vi "Configure All.vi"(8 "error in":errorcluster, 11 "ActorMeter in":refnum<class "ActorMeter.lvclass">) -> (0 "error out":errorcluster, 3 "ActorMeter out":refnum<class "ActorMeter.lvclass">)   [LabVIEW 2014]
uses:
  Implementations/Collector/AverageCollector1D/AverageCollector1D.lvclass
  Implementations/Extractor/MassSpectrumExtractor/MassSpectrumExtractor.lvclass
  <vilib>/ActorFramework/Actor/Actor.lvclass
  StorageService/StorageService.lvclass
  <vilib>/ActorFramework/Message/Message.lvclass
  <vilib>/ActorFramework/Message Enqueuer/Message Enqueuer.lvclass
  Model/Data/MessageToSend.ctl
  ExperimentService/ExperimentService Messages/Set Next Parameter Msg/Set Next Parameter Msg.lvclass
  ExperimentService/ExperimentService.lvclass
  StorageService/StorageService Messages/Register Msg/Register Msg.lvclass
  Model/ReplayData Msg/ReplayData Msg.lvclass
  Hardware/ParameterDevice/ParameterDevice Messages/Get Parameter Msg/Get Parameter Msg.lvclass
  StorageService/StorageService Messages/Notify All Objects Msg/Notify All Objects Msg.lvclass
  ExperimentService/ExperimentService Messages/Write StorageService Msg/Write StorageService Msg.lvclass
  Interfaces/Observable Actor/Observable Actor.lvclass
  Interfaces/Observable Actor/Observable Actor Messages/Add On Event Message Msg/Add On Event Message Msg.lvclass
  Interfaces/Observable Actor/Read Data Msg/Read Data Msg.lvclass
  <vilib>/ActorFramework/Message Enqueuer/Message Priority.ctl
  Implementations/Hardware/Simulated Hardware/ReadoutDevice/Simulated Oscilloscope/Simulated Oscilloscope.lvclass
  Implementations/Hardware/Real Hardware/ReadoutDevice/Agilent DSO-X 3032A/Agilent DSO-X 3032A.lvclass
  <vilib>/Utility/sysdir.llb/System Directory Type.ctl
  Processor/AbstractProcessor1D/AbstractProcessor1D.lvclass
  Implementations/Hardware/Simulated Hardware/ReadoutDevice/Simulated Videocamera/Simulated Videocamera.lvclass
  Implementations/Hardware/Simulated Hardware/ParameterDevice/Simulated ParameterDevice/Simulated ParameterDevice.lvclass
  Processor/AbstractProcessor2D/AbstractProcessor2D.lvclass
  Implementations/Collector/AverageCollector2D/AverageCollector2D.lvclass
  Implementations/Extractor/ImagingExtractor/ImagingExtractor.lvclass
  Extractor/AbstractExtractor/AbstractExtractor.lvclass
  Implementations/Hardware/Real Hardware/ReadoutDevice/Videoscan/Videoscan.lvclass
  SimpleExperimentService/SimpleExperimentService.lvclass
  Implementations/Hardware/Real Hardware/ParameterDevice/SolarSystems M266/SolarSystems M266.lvclass
  Implementations/Hardware/Real Hardware/ParameterDevice/Stepper3D/Stepper3D.lvclass
  ActorMeter.lvclass
  Implementations/Hardware/Real Hardware/ParameterDevice/SolarSystems M266 Old/SolarSystems M266 Old.lvclass
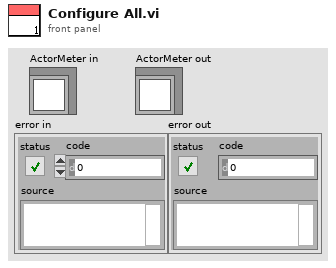
[diagram p1: front panel]
types:
  T1 = typedef "MessageToSend.ctl" = cluster{"Enqueuer":refnum<class "Message Enqueuer.lvclass">, "Message":refnum<class "Message.lvclass">}
  T2 = cluster{"Enqueuer":refnum<class "Message Enqueuer.lvclass">, "Message":refnum<class "ReplayData Msg.lvclass">}
  T3 = typedef "Actor Framework.lvlib/Message Enqueuer.lvclass/Message Priority.ctl" = enum16{"Low", "Normal", "High"}
  T4 = typedef "System Directory Type.ctl" = i32
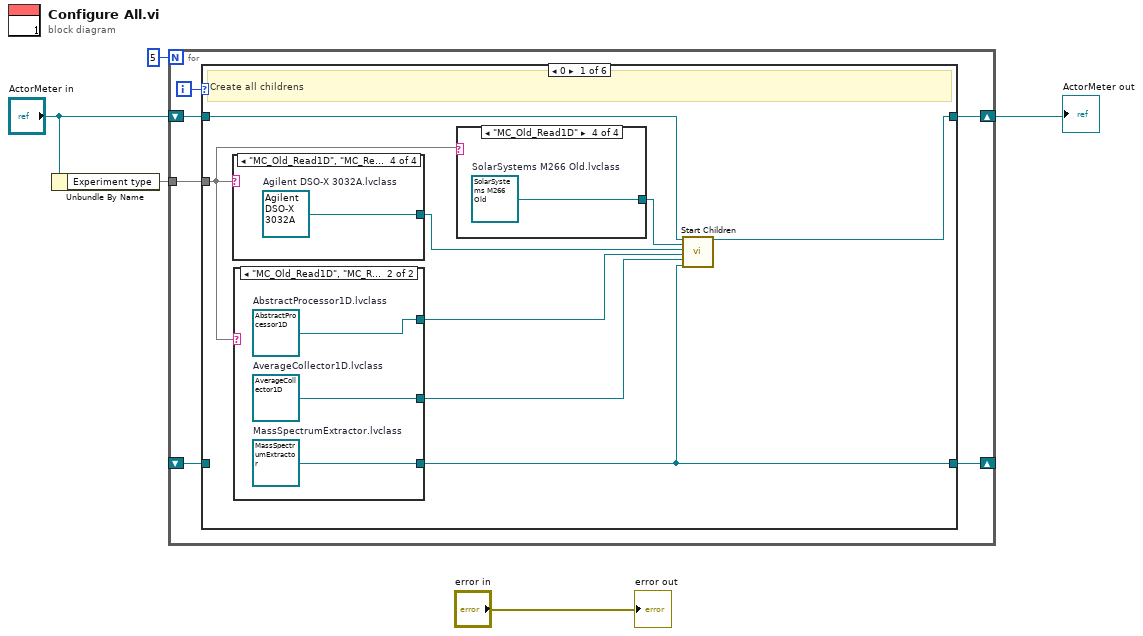
[diagram p0: block diagram]
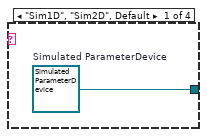
[diagram p2: hidden frame]
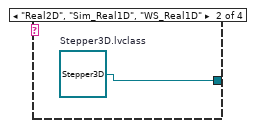
[diagram p3: hidden frame]
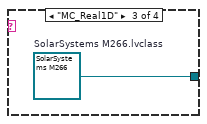
[diagram p4: hidden frame]
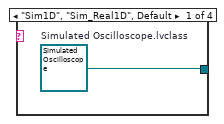
[diagram p5: hidden frame]
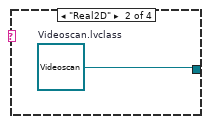
[diagram p6: hidden frame]
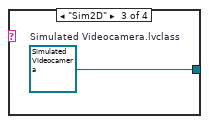
[diagram p7: hidden frame]
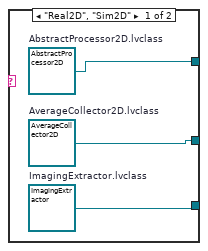
[diagram p8: hidden frame]
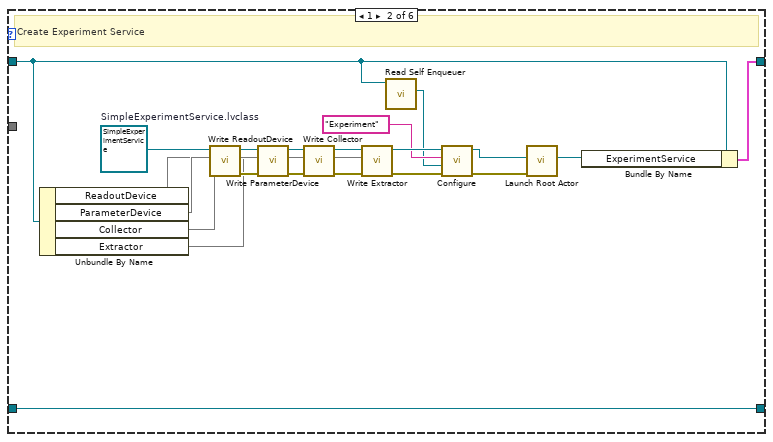
[diagram p9: hidden frame]
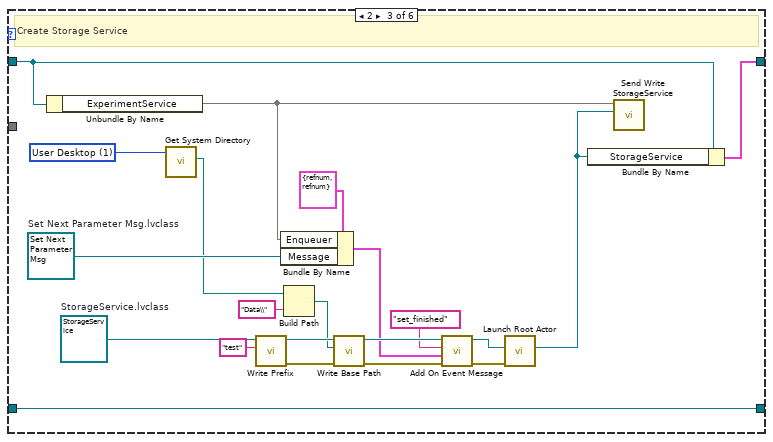
[diagram p10: hidden frame]
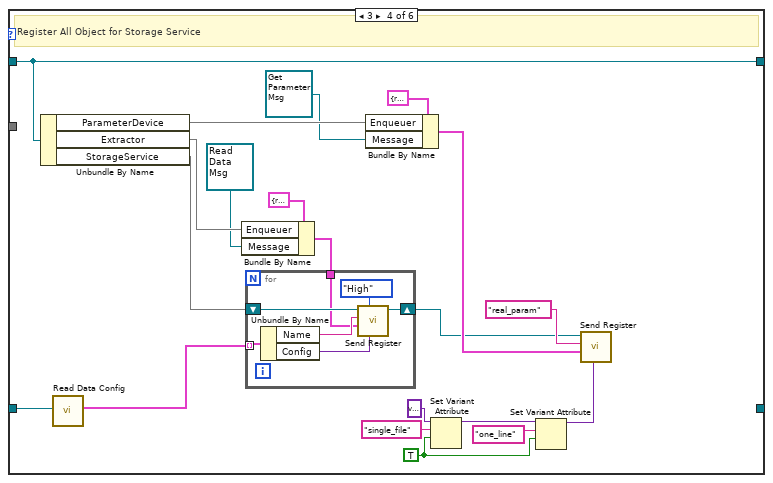
[diagram p11: hidden frame]
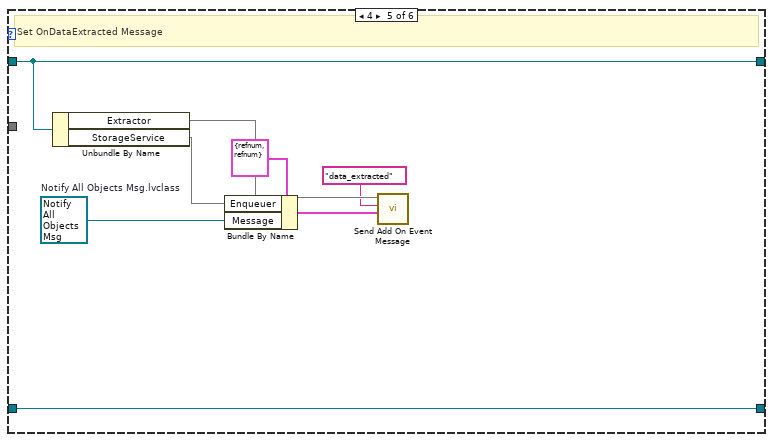
[diagram p12: hidden frame]
diagram:
  n1 = Unbundle By Name("ActorMeter in") -> ("Experiment type"=w1)
  n2 = for {
    N: 5 -> [_]
    shift-right: [w10] -> w3
    shift-left: "ActorMeter in" -> [w11]
    shift-right: [w8] -> _
    shift-left: _ -> [w7]
    tunnel: w1 -> [w6]
    i -> [w9]
    n3 = case shown="0" w9 {
      tunnel: w11 -> [w19 w35 w69 w95 w110 w111]
      tunnel: [w18 w46 w68 w95 w110 w111] -> w10
      tunnel: [w12 w45 w55 _ w103 _] -> w8
      tunnel: w7 -> [_ w45 w55 w80 w103 _]
      tunnel: w6 -> [w17 _ _ _ _ _]
      frame 0 {
        # "Create all childrens"
        n4 = case shown="\"MC_Old_Read1D\", \"MC_Real1D\", \"WS_Real1D\"" w17 {
          tunnel: [w24 w25 w26 w27] -> w15
          frame "Sim1D", "Sim_Real1D", Default {
            w24 = refnum<class "Simulated Oscilloscope.lvclass"> refnum  # Simulated Oscilloscope.lvclass
          }
          frame "Real2D" {
            w25 = refnum<class "Videoscan.lvclass"> refnum  # Videoscan.lvclass
          }
          frame "Sim2D" {
            w26 = refnum<class "Simulated Videocamera.lvclass"> refnum  # Simulated Videocamera.lvclass
          }
          frame "MC_Old_Read1D", "MC_Real1D", "WS_Real1D" {
            w27 = refnum<class "Agilent DSO-X 3032A.lvclass"> refnum  # Agilent DSO-X 3032A.lvclass
          }
        }
        n5 = case shown="\"MC_Old_Read1D\", \"MC_Real1D\", \"Sim1D\", \"Sim_Real1D\", \"WS_Real1D\", Default" w17 {
          tunnel: [w30 w33] -> w14
          tunnel: [w29 w31] -> w13
          tunnel: [w28 w32] -> w12
          frame "Real2D", "Sim2D" {
            w28 = refnum<class "ImagingExtractor.lvclass"> refnum  # ImagingExtractor.lvclass
            w29 = refnum<class "AverageCollector2D.lvclass"> refnum  # AverageCollector2D.lvclass
            w30 = refnum<class "AbstractProcessor2D.lvclass"> refnum  # AbstractProcessor2D.lvclass
          }
          frame "MC_Old_Read1D", "MC_Real1D", "Sim1D", "Sim_Real1D", "WS_Real1D", Default {
            w32 = refnum<class "MassSpectrumExtractor.lvclass"> refnum  # MassSpectrumExtractor.lvclass
            w31 = refnum<class "AverageCollector1D.lvclass"> refnum  # AverageCollector1D.lvclass
            w33 = refnum<class "AbstractProcessor1D.lvclass"> refnum  # AbstractProcessor1D.lvclass
          }
        }
        n6 = case shown="\"MC_Old_Read1D\"" w17 {
          tunnel: [w20 w21 w22 w23] -> w16
          frame "Sim1D", "Sim2D", Default {
            w20 = refnum<class "Simulated ParameterDevice.lvclass"> refnum  # Simulated ParameterDevice
          }
          frame "Real2D", "Sim_Real1D", "WS_Real1D" {
            w21 = refnum<class "Stepper3D.lvclass"> refnum  # Stepper3D.lvclass
          }
          frame "MC_Real1D" {
            w22 = refnum<class "SolarSystems M266.lvclass"> refnum  # SolarSystems M266.lvclass
          }
          frame "MC_Old_Read1D" {
            w23 = refnum<class "SolarSystems M266 Old.lvclass"> refnum  # SolarSystems M266 Old.lvclass
          }
        }
        n7 = call "Start Children.vi"("ActorMeter in"=w19, "ParameterDevice.lvclass"=w16, "ReadoutDevice.lvclass"=w15, "AbstractProcessor.lvclass"=w14, "AbstractCollector.lvclass"=w13, "AbstractExtractor.lvclass"=w12) -> ("ActorMeter out"=w18:refnum<class "ActorMeter.lvclass">)  [unwired: 13 in]
      }
      frame 1 {
        w44 = refnum<class "SimpleExperimentService.lvclass"> refnum  # SimpleExperimentService.lvclass
        # "Create Experiment Service"
        n8 = Unbundle By Name(w35) -> ("ReadoutDevice"=w50, "ParameterDevice"=w51, "Collector"=w49, "Extractor"=w41)
        n9 = call "Write ReadoutDevice.vi"("ReadoutDevice"=w50, "ExperimentService in"=w44) -> ("error out"=w52:errorcluster, "ExperimentService out"=w47:refnum<class "SimpleExperimentService.lvclass">)  [unwired: 8 in]
        n10 = call "Write ParameterDevice.vi"("error in (no error)"=w52, "Parameter Device"=w51, "ExperimentService in"=w47) -> ("error out"=w53:errorcluster, "ExperimentService out"=w48:refnum<class "SimpleExperimentService.lvclass">)  [unwired: 7 in]
        n11 = call "Write Collector.vi"("error in (no error)"=w53, "Collector"=w49, "ExperimentService in"=w48) -> ("error out"=w42:errorcluster, "ExperimentService out"=w43:refnum<class "SimpleExperimentService.lvclass">)  [unwired: 7 in]
        n12 = call-dynamic "Write Extractor.vi"("error in (no error)"=w42, "Extractor"=w41, "ExperimentService in"=w43) -> ("error out"=w39:errorcluster, "ExperimentService out"=w40:refnum<class "SimpleExperimentService.lvclass">)  [unwired: 7 in]
        n13 = call <vilib>:"Read Self Enqueuer.vi"("Actor"=w35) -> ("Self Enqueuer"=w34:refnum<class "Message Enqueuer.lvclass">)  [unwired: 10 in]
        n14 = call-dynamic "Configure.vi"("error in (no error)"=w39, "ActorMeter Enqueuer"=w34, "Name"="Experiment", "Viewable Actor in"=w40) -> ("error out"=w37:errorcluster, "Viewable Actor out"=w38:refnum<class "SimpleExperimentService.lvclass">)  [unwired: 6 in]
        n15 = call <vilib>:"Launch Root Actor.vi"("error in (no error)"=w37, "Actor"=w38) -> ("Actor's Enqueuer"=w54:refnum<class "Message Enqueuer.lvclass">)  [unwired: 8 in, 1 out]
        n16 = Bundle By Name(cluster=w35, "ExperimentService"=w54) -> (w46:cluster{})
      }
      frame 2 {
        w57 = T4 1 items=["User Home"=0, "User Desktop"=1, "User Documents"=2, "User Application Data"=3, "User Preferences"=4, "User Temporary"=5, "Public Documents"=6, "Public Application Data"=7, "Public Preferences"=8, "Public Cache"=13, "System Core Libraries"=9, "System Installed Libraries"=10, "Application Files"=11, "Boot Volume Root"=12] ("system directory type")
        w75 = refnum<class "Set Next Parameter Msg.lvclass"> refnum  # Set Next Parameter Msg.lvclass
        w72 = refnum<class "StorageService.lvclass"> refnum  # StorageService.lvclass
        # "Create Storage Service"
        n17 = Unbundle By Name(w69) -> ("ExperimentService"=w67)
        n18 = call <vilib>:"Get System Directory.vi"("system directory type"=w57) -> ("system directory"=w56:path)  [unwired: 10 in]
        n19 = call-dynamic "Write Prefix.vi"("Prefix"="test", "StorageService in"=w72) -> ("error out"=w70:errorcluster, "StorageService out"=w71:refnum<class "StorageService.lvclass">)  [unwired: 8 in]
        n20 = Bundle By Name(cluster=T1 {"Enqueuer"=refnum, "Message"=refnum} ("Message To Send"), "Enqueuer"=w67, "Message"=w75) -> (w59:T1)
        n21 = Build Path(base path=w56, name or relative path="Data\\") -> (appended path=w64:path)
        n22 = call-dynamic "Write Base Path.vi"("error in (no error)"=w70, "Base Path"=w64, "StorageService in"=w71) -> ("error out"=w61:errorcluster, "StorageService out"=w63:refnum<class "StorageService.lvclass">)  [unwired: 7 in]
        n23 = call "Add On Event Message.vi"("error in (no error)"=w61, "Message To Send"=w59, "Event"="set_finished", "Observable Actor in"=w63) -> ("error out"=w60:errorcluster, "Observable Actor out"=w62:refnum<class "StorageService.lvclass">)  [unwired: 6 in]
        n24 = call <vilib>:"Launch Root Actor.vi"("error in (no error)"=w60, "Actor"=w62) -> ("Actor's Enqueuer"=w66:refnum<class "Message Enqueuer.lvclass">)  [unwired: 8 in, 1 out]
        n25 = Bundle By Name(cluster=w69, "StorageService"=w66) -> (w68:cluster{})
        n26 = call "Send Write StorageService.vi"("StorageService"=w66, "Message Enqueuer"=w67) -> ()  [unwired: 8 in, 2 out]
      }
      frame 3 {
        w83 = TRUE ("Save to single file")
        # "Register All Object for Storage Service"
        n27 = Unbundle By Name(w95) -> ("ParameterDevice"=w93, "Extractor"=w88, "StorageService"=w77)
        n28 = call-dynamic "Read Data Config.vi"("Observable Actor in"=w80) -> ("Extracted Data Info"=w79:cluster{"Name":string, "Config":variant}[])  [unwired: 8 in, 2 out]
        n29 = Bundle By Name(cluster=T2 {"Enqueuer"=refnum, "Message"=refnum} ("GetData Message"), "Enqueuer"=w88, "Message"=refnum<class "Read Data Msg.lvclass"> refnum ("Observable Actor.lvlib:Read Data Msg.lvclass")) -> (w78:T2)
        n30 = for {
          tunnel: w79 -> [w102] mode=indexing
          tunnel: w78 -> [w97]
          shift-right: [w100] -> w76
          shift-left: w77 -> [w101]
          n31 = Unbundle By Name(w102) -> ("Name"=w99:string, "Config"=w98:variant)
          n32 = call "Send Register.vi"("Save Parameters"=w98, "Message Priority (Normal)"=Message_Priority."High", "GetData Message"=w97, "Name"=w99, "Message Enqueuer"=w101) -> ("Message Enqueuer out"=w100:refnum<class "Message Enqueuer.lvclass">)  [unwired: 5 in, 1 out]
        }
        n33 = Bundle By Name(cluster=T2 {"Enqueuer"=refnum, "Message"=refnum} ("GetData Message"), "Enqueuer"=w93, "Message"=refnum<class "Get Parameter Msg.lvclass"> refnum ("Get Parameter Msg.lvclass")) -> (w90:T2)
        n34 = Set Variant Attribute(Variant=variant ("variant"), name="single_file", value=w83) -> (Variant out=w85:variant)  [unwired: 1 in, 2 out]
        n35 = Set Variant Attribute(Variant=w85, name="one_line", value=w83) -> (Variant out=w82:variant)  [unwired: 1 in, 2 out]
        n36 = call "Send Register.vi"("Save Parameters"=w82, "GetData Message"=w90, "Name"="real_param", "Message Enqueuer"=w76) -> ()  [unwired: 6 in, 2 out]
      }
      frame 4 {
        w107 = refnum<class "Notify All Objects Msg.lvclass"> refnum  # Notify All Objects Msg.lvclass
        # "Set OnDataExtracted Message"
        n37 = Unbundle By Name(w110) -> ("Extractor"=w106, "StorageService"=w108)
        n38 = Bundle By Name(cluster=T1 {"Enqueuer"=refnum, "Message"=refnum} ("Message To Send"), "Enqueuer"=w108, "Message"=w107) -> (w105:T1)
        n39 = call "Send Add On Event Message.vi"("Message To Send"=w105, "Event"="data_extracted", "Message Enqueuer"=w106) -> ()  [unwired: 7 in, 2 out]
      }
      frame Default {
      }
    }
  }
  "ActorMeter out" <- w3
  "error out" <- "error in"
